vi "Read lvsocket.vi"(11 "lvlibretls connection in":refnum<class "lvlibretls connection.lvclass">) -> (2 "lvsocket":u64, 3 "lvlibretls connection out":refnum<class "lvlibretls connection.lvclass">)   [LabVIEW 2016, in "lvlibretls connection.lvclass"]
uses:
  lvlibretls connection.lvclass
  lvlibretls connection.lvclass/lvlibretls connection.ctl
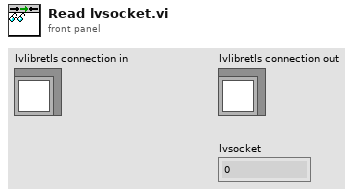
[diagram p1: front panel]
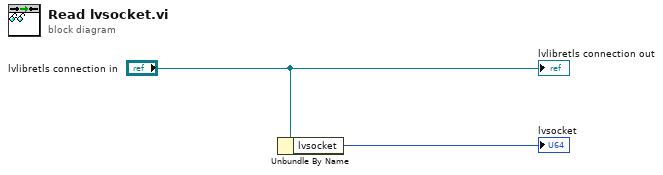
[diagram p0: block diagram]
diagram:
  n1 = Unbundle By Name("lvlibretls connection in") -> ("lvsocket"=→"lvsocket":u64)
  "lvlibretls connection out" <- "lvlibretls connection in"
